vi "EditorFillOrDropRows.vi"(10 "NewRows":i32, 11 "Array in":i32[][](array[numeric])) -> (3 "Array out":i32[][](array[numeric]))   [LabVIEW 2020]
doc: "Takes existing 2D array and new number of rows and fills new rows with 0s or drops some rows from the end"
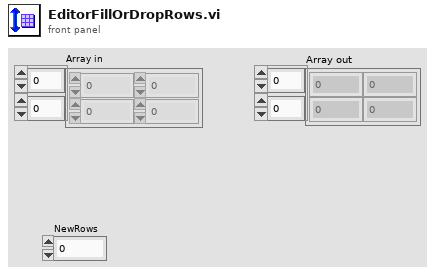
[diagram p1: front panel]
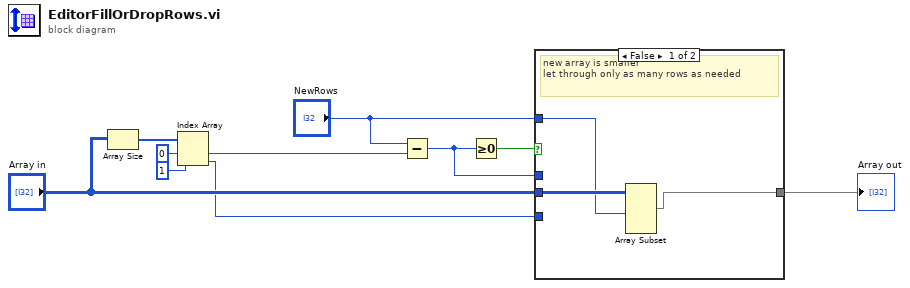
[diagram p0: block diagram]
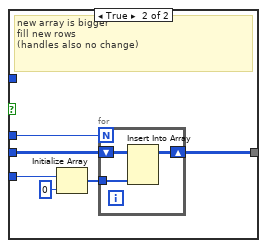
[diagram p2: hidden frame]
diagram:
  n1 = Array Size(array="Array in") -> (size(s)=w6:i32[])
  n2 = Index Array(array=w6, index #1=0 ("index"), index #2=1 ("index")) -> (element #1=w3:i32, element #2=w2:i32)
  n3 = Subtract(x="NewRows", y=w3) -> (x-y=w9:i32)
  n4 = Greater Or Equal To 0?(x=w9) -> (x >= 0?=w8:bool)
  n5 = case shown="False" w8 {
    tunnel: [w11 w18] -> w10
    tunnel: "Array in" -> [w13 w17]
    tunnel: w9 -> [_ w15]
    tunnel: w2 -> [_ w14]
    tunnel: "NewRows" -> [w12 _]
    frame False {
      # "new array is smaller\nlet through only as many rows as needed"
      n6 = Array Subset(array=w13, length (row)=w12) -> (w11:i32[][])  [unwired: 3 in]
    }
    frame True {
      # "new array is bigger\nfill new rows\n(handles also no change)"
      n7 = Initialize Array(w14, 0 ("dimension size")) -> (w19:i32[])
      n8 = for {
        N: w15 -> [_]
        tunnel: w19 -> [w21]
        shift-right: [w20] -> w18
        shift-left: w17 -> [w22]
        n9 = Insert Into Array(array=w22, new element=w21) -> (w20:i32[][])  [unwired: 2 in]
      }
    }
  }
  "Array out" <- w10
